vi "xijk_comma_dot_replacement.vi"(1 "table in":string[](array[string])) -> (0 "table out":string[](array[string]))   [LabVIEW 2009]
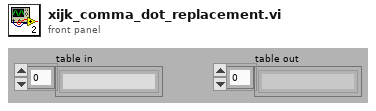
[diagram p1: front panel]
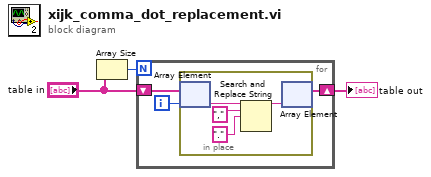
[diagram p0: block diagram]
diagram:
  n1 = Array Size(array="table in") -> (size(s)=w1:i32)
  n2 = for {
    N: w1 -> [_]
    shift-right: [w4] -> w3
    shift-left: "table in" -> [w6]
    i -> [w5]
    n3 = in-place {
      n4 = in-place-array #1(w6, w5) -> (w8:string)
      n5 = Search and Replace String(input string=w8, search string="," ("chaîne recherchée"), replace string="." ("chaîne de remplacement (\"\")")) -> (result string=w7:string)  [unwired: 1 in, 7 out]
      n6 = in-place-array #1(w7) -> (w4:string[])  [unwired: 1 out]
    }
  }
  "table out" <- w3
